vi "Lettura Proximity_fin.vi"() -> ()   [LabVIEW 2021]
uses:
  <vilib>/DAQmx/read.llb/DAQmx Read (Analog Wfm 1Chan NSamp).vi
  <vilib>/Analysis/baseanly.llb/Mean (DBL).vi
  <vilib>/DAQmx/configure/timing.llb/DAQmx Timing (Sample Clock).vi
  <vilib>/DAQmx/miscellaneous.llb/DAQmx Fill In Error Info.vi
  <vilib>/Utility/file.llb/Write Delimited Spreadsheet (DBL).vi
  <vilib>/Analysis/NI_AALBase.lvlib
panel:
  out "Minimo":dbl
  out "Massimo":dbl
  out "Deviazione Standard":dbl format="%0.2f"
  out "Media":dbl format="%0.2f"
  in  "File txt Distanza":path
  out "Distanza":dbl[](graph)
  out "Segnale Proximity":waveform(dbl)(graph)
  out "num campioni":dbl
  in  "File txt Tensione":path
  in  "SAVE":bool
  in  "Frequenza":dbl=5000.0 format="%0.2p"
  in  "Durata":dbl=0.1 format="%.2p"
  in  "STOP":bool
  out "current time":timestamp
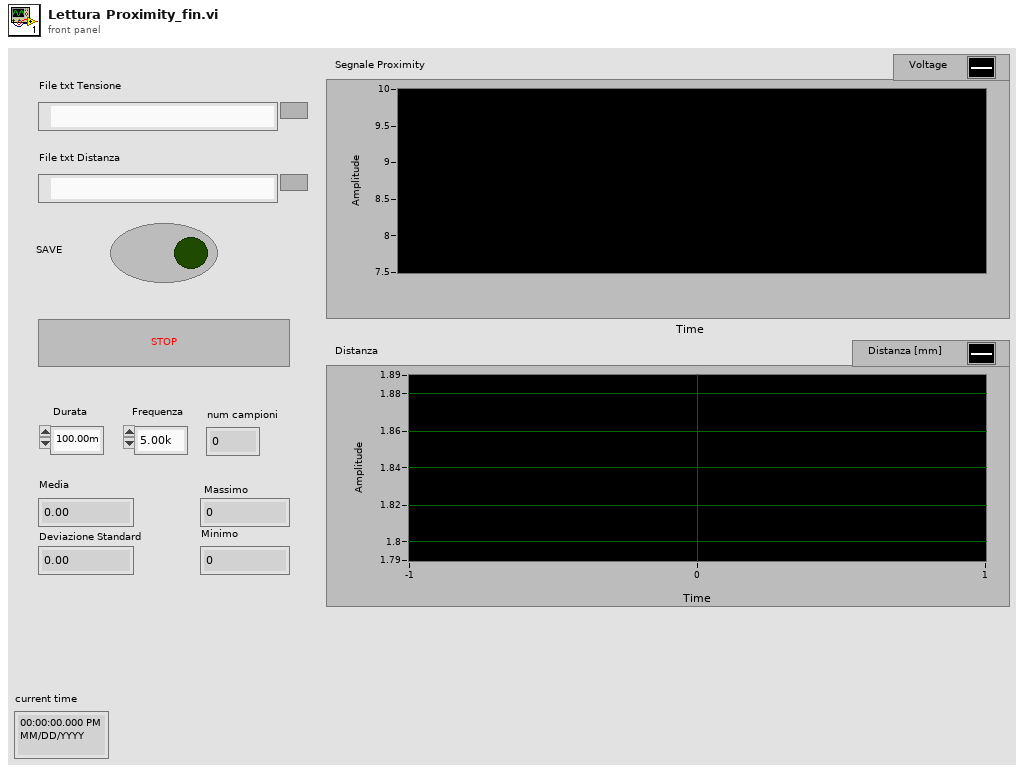
[diagram p1: front panel]
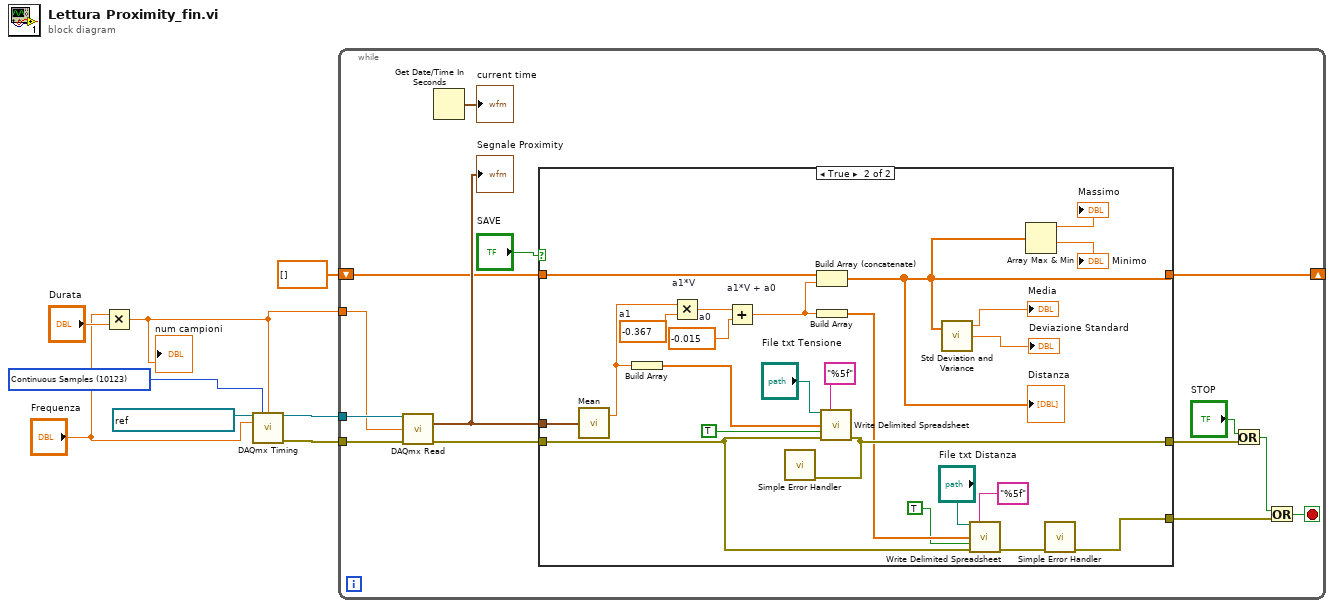
[diagram p0: block diagram]
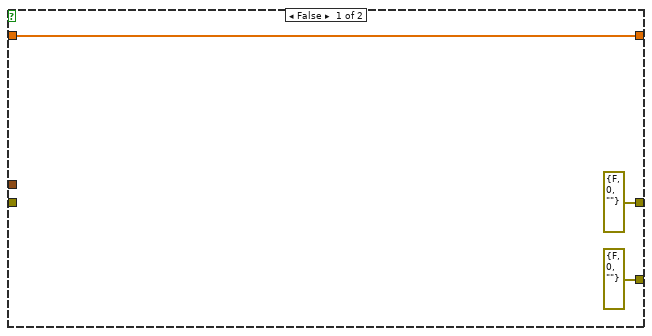
[diagram p2: hidden frame]
diagram:
  w4 = 10123 items=["Finite Samples"=10178, "Continuous Samples"=10123, "Hardware Timed Single Point"=12522] ("sample mode")
  n1 = Multiply(x="Frequenza", y="Durata") -> (x*y=w5:dbl)
  "num campioni" <- w5
  n2 = call-poly <vilib>:"DAQmx Timing.vi"("task/channels in"=refnum<k21> "MyVoltageTask", "sample mode"=w4, "samples per channel"=w5, "rate"="Frequenza") -> ("task out"=w8:refnum<k21>, "error out"=w3:errorcluster)  [unwired: 10 in]
  n3 = while {
    tunnel: w8 -> [w20]
    tunnel: w5 -> [w19]
    tunnel: w3 -> [w18]
    shift-right: [w13] -> _
    shift-left: dbl[] [] -> [w12]
    stop <- w9 stop-if-true
    n4 = call-poly <vilib>:"DAQmx Read.vi"("task/channels in"=w20, "number of samples per channel"=w19, "error in"=w18) -> ("data"=w16:waveform(dbl), "error out"=w15:errorcluster)  [unwired: 10 in, 1 out]
    "Segnale Proximity" <- w16
    n5 = Get Date/Time In Seconds() -> (seconds since 1Jan1904=→"current time":timestamp)
    n6 = case shown="True" "SAVE" {
      tunnel: [errorcluster {"status"=FALSE, "code"=0, "source"=""} ("error IO") w48] -> w21
      tunnel: w16 -> [_ w47]
      tunnel: w15 -> [_ w40]
      tunnel: [w24 w28] -> w13
      tunnel: w12 -> [w24 w31]
      tunnel: [errorcluster {"status"=FALSE, "code"=0, "source"=""} ("error out") w38] -> w11
      frame False {
      }
      frame True {
        w33 = -0.015  # a0
        w34 = -0.367  # a1
        n7 = call-poly <vilib>:"Mean.vi"("X"=w47) -> ("mean"=w35:dbl)  [unwired: 1 out]
        n8 = Build Array(w35) -> (w44:dbl[])
        n9 = Multiply "a1*V"(x=w35, y=w34) -> (x*y=w36:dbl)
        n10 = Add "a1*V + a0"(x=w36, y=w33) -> (x+y=w32:dbl)
        n11 = Build Array (concatenate)(w31, w32) -> (w28:dbl[])
        "Distanza" <- w28
        n12 = Build Array(w32) -> (w43:dbl[])
        n13 = call-poly <vilib>:"Write Delimited Spreadsheet.vi"("file path (dialog if empty)"="File txt Tensione", "format (%.3f)"="%5f", "1D data"=w44, "append to file? (new file:F)"=TRUE, "error in (no error)"=w40) -> ("error out"=w48:errorcluster)  [unwired: 9 in, 1 out]
        n14 = call <vilib>:"Simple Error Handler.vi"("error in (no error)"=w48) -> ()  [unwired: 4 in, 5 out]
        n15 = call <vilib>:"Std Deviation and Variance.vi"("X"=w28) -> ("mean"=→"Media":dbl, "standard deviation"=→"Deviazione Standard":dbl)  [unwired: 1 in, 1 out]
        n16 = call-poly <vilib>:"Write Delimited Spreadsheet.vi"("file path (dialog if empty)"="File txt Distanza", "format (%.3f)"="%5f", "1D data"=w43, "append to file? (new file:F)"=TRUE, "error in (no error)"=w40) -> ("error out"=w39:errorcluster)  [unwired: 9 in, 1 out]
        n17 = Array Max & Min(array=w28) -> (max value=→"Massimo":dbl, min value=→"Minimo":dbl)  [unwired: 2 out]
        n18 = call <vilib>:"Simple Error Handler.vi"("error in (no error)"=w39) -> ("error out"=w38:errorcluster)  [unwired: 4 in, 4 out]
      }
    }
    n19 = Or(x="STOP", y=w21) -> (x .or. y?=w10:bool)
    n20 = Or(x=w10, y=w11) -> (x .or. y?=w9:bool)
  }
